vi "Last_modified_date.vi"(0 "Update Now":bool) -> (1 "RevisionString":string, 2 "BasesvnRevision":u32)   [LabVIEW 2011]
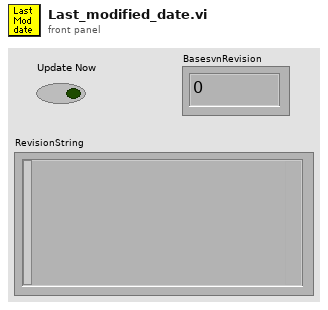
[diagram p1: front panel]
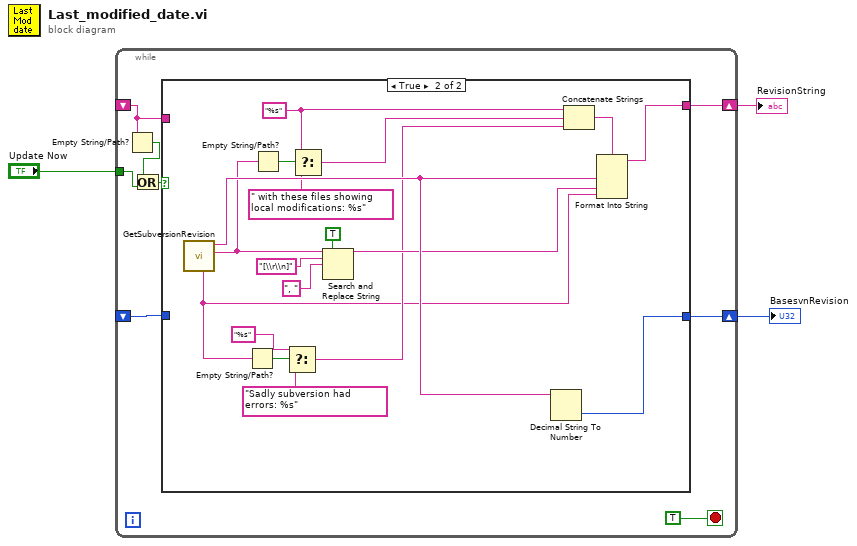
[diagram p0: block diagram]
diagram:
  n1 = while {
    shift-right: [w11] -> w3
    shift-left: _ -> [w10]
    shift-right: [w8] -> w2
    shift-left: _ -> [w7]
    tunnel: "Update Now" -> [w5]
    stop <- TRUE stop-if-true
    n2 = Empty String/Path?(string/path=w10) -> (empty?=w4:bool)
    n3 = Or(x=w4, y=w5) -> (x .or. y?=w6:bool)
    n4 = case shown="True" w6 {
      tunnel: [w13 w29] -> w11
      tunnel: w10 -> [w13 _]
      tunnel: [w12 w31] -> w8
      tunnel: w7 -> [w12 _]
      frame False {
      }
      frame True {
        w21 = "%s" ("format string")
        n5 = call "GetSubversionRevision.vi"() -> ("LocalModifications"=w25:string, "OverallRevision"=w30:string, "standard error"=w15:string)  [unwired: 6 in, 3 out]
        n6 = Empty String/Path?(string/path=w15) -> (empty?=w18:bool)
        n7 = Empty String/Path?(string/path=w25) -> (empty?=w24:bool)
        n8 = Select(t="%s" ("format string"), s=w18, f="Sadly subversion had errors: %s" ("format string")) -> (s? t:f=w16:string)
        n9 = Select(t=w21, s=w24, f=" with these files showing local modifications: %s" ("format string")) -> (s? t:f=w22:string)
        n10 = Search and Replace String(replace all?=TRUE ("replace all? (F)"), input string=w25, search string="[\\r\\n]", replace string=", " ("replace string (\"\")")) -> (result string=w28:string)  [unwired: 4 in, 3 out]
        n11 = Decimal String To Number(string=w30) -> (number=w31:i32)  [unwired: 2 in, 1 out]
        n12 = Concatenate Strings(w21, w22, w16) -> (w20:string)
        n13 = Format Into String(format string=w20, w30, w28, w15) -> (resulting string=w29:string)  [unwired: 2 in, 1 out]
      }
    }
  }
  "RevisionString" <- w3
  "BasesvnRevision" <- w2
